vi "Mix.vi"() -> ()   [LabVIEW 2011]
panel:
  out "Waveform Graph":cluster{dbl, dbl, dbl[]}[](graph)
  # "334AB ALEXANDRESCU Anda\nMixaj"
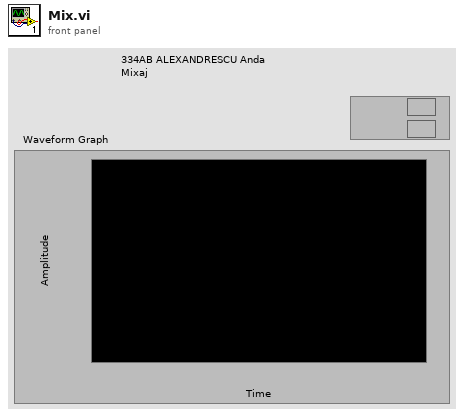
[diagram p1: front panel]
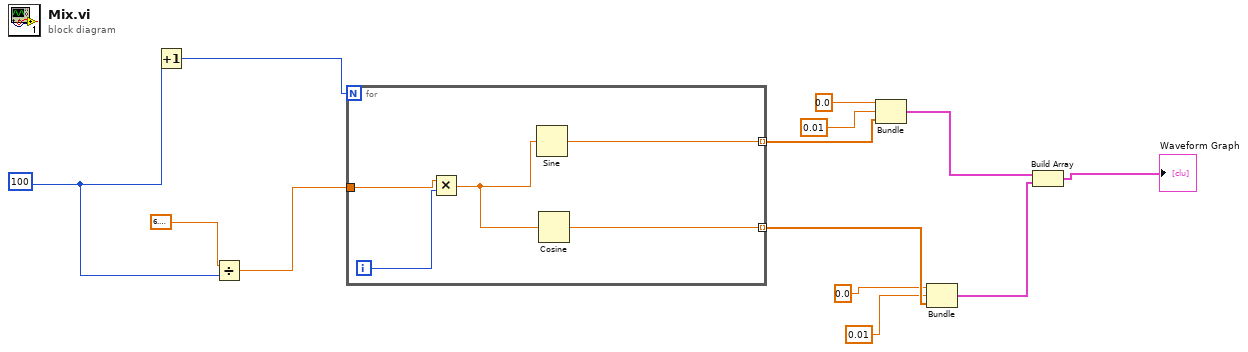
[diagram p0: block diagram]
diagram:
  w11 = 100
  n1 = Increment(x=w11) -> (x+1=w13:i32)
  n2 = Divide(x=6.283185307179586, y=w11) -> (x/y=w10:dbl)
  n3 = for {
    N: w13 -> [_]
    tunnel: w10 -> [w17]
    tunnel: [w15] -> w6 mode=indexing
    tunnel: [w14] -> w3 mode=indexing
    i -> [w18]
    n4 = Multiply(x=w17, y=w18) -> (x*y=w16:dbl)
    n5 = Sine(x=w16) -> (sin(x)=w14:dbl)
    n6 = Cosine(x=w16) -> (cos(x)=w15:dbl)
  }
  n7 = Bundle(0.0, 0.01, w3) -> (w2:cluster{dbl, dbl, dbl[]})  [unwired: 1 in]
  n8 = Bundle(0.0, 0.01, w6) -> (w1:cluster{dbl, dbl, dbl[]})  [unwired: 1 in]
  n9 = Build Array(w2, w1) -> (→"Waveform Graph":cluster{dbl, dbl, dbl[]}[])
